vi "HEWH RLT Cutout Checker Pulse Logic.vi"(7 "Previous Full Cutout Value":bool, 8 "Error In":errorcluster, 10 "Cut In Timer (Over)":bool, 11 "Cut Out Timer (Over)":bool) -> (0 "Error Out":errorcluster, 3 "Full Cutout?":bool)   [LabVIEW 2023]
panel:
  out "Cut Out Condition":bool
  out "Cut In Condition":bool
  out "Heat Pulse Condition":bool
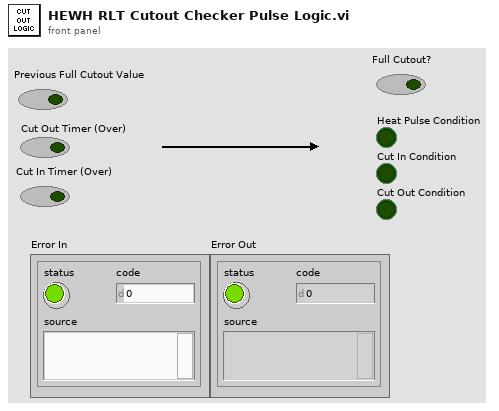
[diagram p1: front panel]
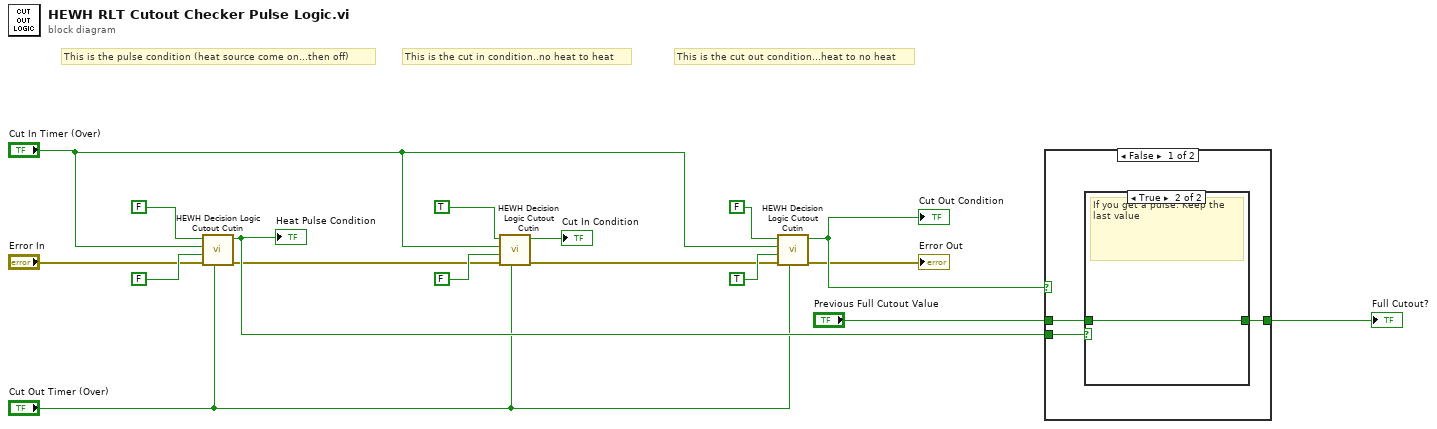
[diagram p0: block diagram]
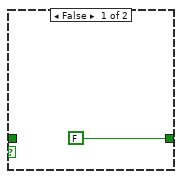
[diagram p2: hidden frame]
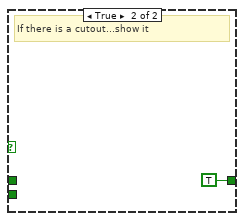
[diagram p3: hidden frame]
diagram:
  # "This is the cut out condition...heat to no heat"
  # "This is the cut in condition..no heat to heat"
  # "This is the pulse condition (heat source come on...then off)"
  n1 = call "HEWH Decision Logic Cutout Cutin.vi"("Cut Out Timer (Over)"="Cut Out Timer (Over)", "Error In"="Error In", "Bottom"=FALSE ("x"), "Cut In Timer (Over)"="Cut In Timer (Over)", "Top"=FALSE ("y")) -> ("Error Out"=w4:errorcluster, "Output"=w15:bool)  [unwired: 5 in]
  "Heat Pulse Condition" <- w15
  n2 = call "HEWH Decision Logic Cutout Cutin.vi"("Cut Out Timer (Over)"="Cut Out Timer (Over)", "Error In"=w4, "Bottom"=FALSE ("y"), "Cut In Timer (Over)"="Cut In Timer (Over)", "Top"=TRUE ("y")) -> ("Error Out"=w3:errorcluster, "Output"=→"Cut In Condition":bool)  [unwired: 5 in]
  n3 = call "HEWH Decision Logic Cutout Cutin.vi"("Cut Out Timer (Over)"="Cut Out Timer (Over)", "Error In"=w3, "Bottom"=TRUE ("y"), "Cut In Timer (Over)"="Cut In Timer (Over)", "Top"=FALSE ("y")) -> ("Error Out"=→"Error Out":errorcluster, "Output"=w5:bool)  [unwired: 5 in]
  "Cut Out Condition" <- w5
  n4 = case shown="False" w5 {
    tunnel: [w20 TRUE] -> w16
    tunnel: w15 -> [w19 _]
    tunnel: "Previous Full Cutout Value" -> [w18 _]
    frame False {
      n5 = case shown="True" w19 {
        tunnel: [FALSE w22] -> w20
        tunnel: w18 -> [_ w22]
        frame False {
        }
        frame True {
          # "If you get a pulse. Keep the last value"
        }
      }
    }
    frame True {
      # "If there is a cutout...show it"
    }
  }
  "Full Cutout?" <- w16
